vi "Untitled 1.vi"   [LabVIEW 2015]
types:
  T1 = typedef "WPI_JoystickDevRef.ctl" = cluster{"Device":T2}
  T2 = typedef "WPI_JoystickDeviceEnum.ctl" = enum16{"USB 0", "USB 1", "USB 2", "USB 3", "USB 4", "USB 5"}
  T3 = cluster{"Axes[0]":dbl, "Axes[1]":dbl, "Axes[2]":dbl, "Axes[3]":dbl, "Axes[4]":dbl, "Axes[5]":dbl, "Axes[6]":dbl, "Axes[7]":dbl, "Axes[8]":dbl}
  T4 = cluster{"Buttons[0]":bool, "Buttons[1]":bool, "Buttons[2]":bool, "Buttons[3]":bool, "Buttons[4]":bool, "Buttons[5]":bool, "Buttons[6]":bool, "Buttons[7]":bool, "Buttons[8]":bool}
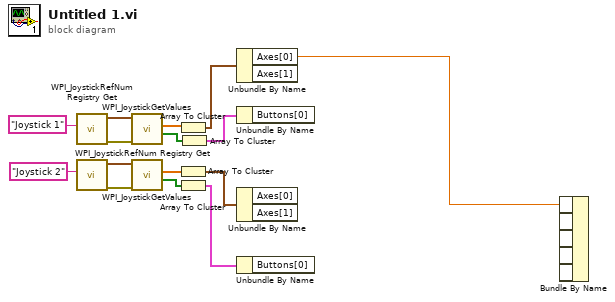
[diagram p0: block diagram]
diagram:
  n1 = call <vilib>:"WPI_JoystickRefNum Registry Get.vi"("refnum name"="Joystick 1") -> ("error out"=w14:errorcluster, "JoystickDevRef"=w13:T1)  [unwired: 9 in]
  n2 = call <vilib>:"WPI_JoystickRefNum Registry Get.vi"("refnum name"="Joystick 2") -> ("error out"=w11:errorcluster, "JoystickDevRef"=w10:T1)  [unwired: 9 in]
  n3 = call <vilib>:"WPI_JoystickGetValues.vi"("error in (no error)"=w14, "JoystickDevRef"=w13) -> ("Buttons"=w8:bool[], "Axes"=w9:dbl[])  [unwired: 5 in, 3 out]
  n4 = call <vilib>:"WPI_JoystickGetValues.vi"("error in (no error)"=w11, "JoystickDevRef"=w10) -> ("Buttons"=w6:bool[], "Axes"=w7:dbl[])  [unwired: 5 in, 3 out]
  n5 = Array To Cluster(array=w9) -> (cluster=w5:T3)
  n6 = Array To Cluster(array=w7) -> (cluster=w3:T3)
  n7 = Array To Cluster(array=w6) -> (cluster=w2:T4)
  n8 = Array To Cluster(array=w8) -> (cluster=w4:T4)
  n9 = Unbundle By Name(w5) -> ("Axes[0]"=w1:dbl)  [unwired: 1 out]
  n10 = Unbundle By Name(w4) -> ()  [unwired: 1 out]
  n11 = Unbundle By Name(w3) -> ()  [unwired: 2 out]
  n12 = Unbundle By Name(w2) -> ()  [unwired: 1 out]
  n13 = Bundle By Name(w1) -> ()  [unwired: 5 in, 1 out]
